vi "OpenMotor.vi"(7 "EnableMotor?(T)":bool=TRUE, 8 "Error In":errorcluster, 9 "CAN ID":u32=1, 10 "MotorType":T1, 11 "USB CAN VISA resource name":refnum<visa-resource-name>="ASRL3::INSTR") -> (0 "Error Out":errorcluster, 3 "Reference Out":T2={"VISA resource name"="", "MotorType"=enum."AK80-64", "CAN ID"=1})   [LabVIEW 2019, in "CubeMarsBLDClib.lvlib"]
uses:
  CubeMarsBLDClib.lvlib
  Reference.ctl
  MotorType.ctl
  MotorParameters.ctl
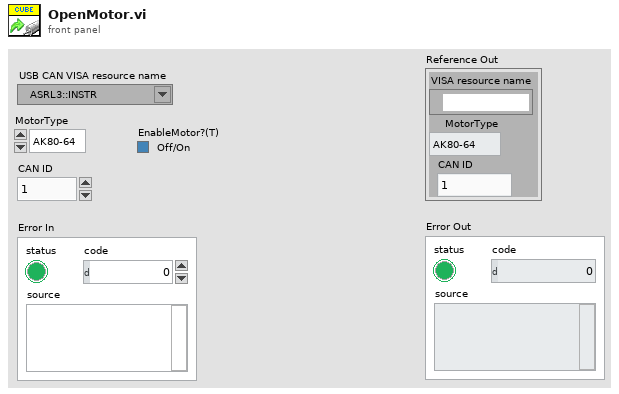
[diagram p1: front panel]
types:
  T1 = typedef "CubeMarsBLDClib.lvlib/MotorType.ctl" = enum16{"AK80-64", "AK80-9", "AK80-8", "AK80-6", "AK70-10", "AK60-6", "AK10-9"}
  T2 = typedef "CubeMarsBLDClib.lvlib/Reference.ctl" = cluster{"VISA resource name":refnum<visa-resource-name>, "MotorType":T1, "CAN ID":u32}
  T3 = typedef "CubeMarsBLDClib.lvlib/MotorParameters.ctl" = cluster{"Position(rad)":dbl, "Speed(rad/s)":dbl, "Kp":dbl, "Kd":dbl, "Torque (N.M)":dbl}
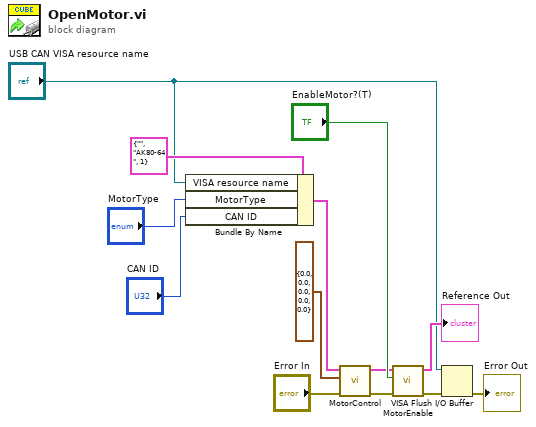
[diagram p0: block diagram]
diagram:
  n1 = Bundle By Name(cluster=T2 {"VISA resource name"="", "MotorType"=enum."AK80-64", "CAN ID"=1} ("Reference out"), "VISA resource name"="USB CAN VISA resource name", "MotorType"="MotorType", "CAN ID"="CAN ID") -> (w7:T2)
  n2 = call "MotorControl.vi"("error in"="Error In", "ValueIn"=T3 {"Position(rad)"=0.0, "Speed(rad/s)"=0.0, "Kp"=0.0, "Kd"=0.0, "Torque (N.M)"=0.0}, "Reference In"=w7) -> ("error out"=w8:errorcluster, "Reference Out"=w5:T2)  [unwired: 6 in, 1 out]
  n3 = call "MotorEnable.vi"("Error In"=w8, "Enable?(F)"="EnableMotor?(T)", "Reference In"=w5) -> ("Error Out"=w3:errorcluster, "Reference Out"=→"Reference Out":T2)  [unwired: 7 in]
  n4 = VISA Flush I/O Buffer(VISA resource name="USB CAN VISA resource name", error in (no error)=w3) -> (error out=→"Error Out":errorcluster)  [unwired: 1 in, 1 out]
